vi "Juk3box_os.vi"() -> ()   [LabVIEW 2016]
uses:
  <vilib>/NXT/Block Support/NXT_InputPort.ctl
  <vilib>/NXT/Block Support/NXT_OutputPort.ctl
  <vilib>/NXT/Dual Mode Library/Sensors/Touch_Pressed.vi
  <vilib>/NXT/NXTIO Xnodes/NXTIONodeSubVIs/NXTMoveMotors.vi
  <vilib>/NXT/Dual Mode Library/Waits/Wait_Num.vi
  <vilib>/NXT/NXTIO Xnodes/NXTIONodeSubVIs/NXTStopMotors.vi
  <vilib>/NXT/Dual Mode Library/Sensors/EV3_Color_Color.vi
  <vilib>/NXT/NXTIO Xnodes/AddressXNode/NXTIOAddress.xnode
  <vilib>/NXT/NXTIO Xnodes/NXTIOXNode/NXTIO.xnode
  <vilib>/NXT/Subs/LVHSConnector.ctl
  <vilib>/NXT/LegoClasses/BrickReference/BrickReference.lvclass
panel:
  in  "Stop":bool
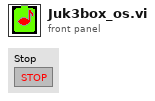
[diagram p1: front panel]
types:
  T1 = typedef "NXT_OutputPort.ctl" = u8
  T2 = typedef "NXT_InputPort.ctl" = u32
  T3 = typedef "LVHSConnector.ctl" = refnum<class "BrickReference.lvclass">
  T4 = typedef "ColorSensorColors.ctl" = enum16{"No Color", "Black", "Blue", "Green", "Yellow", "Red", "White", "Brown"}
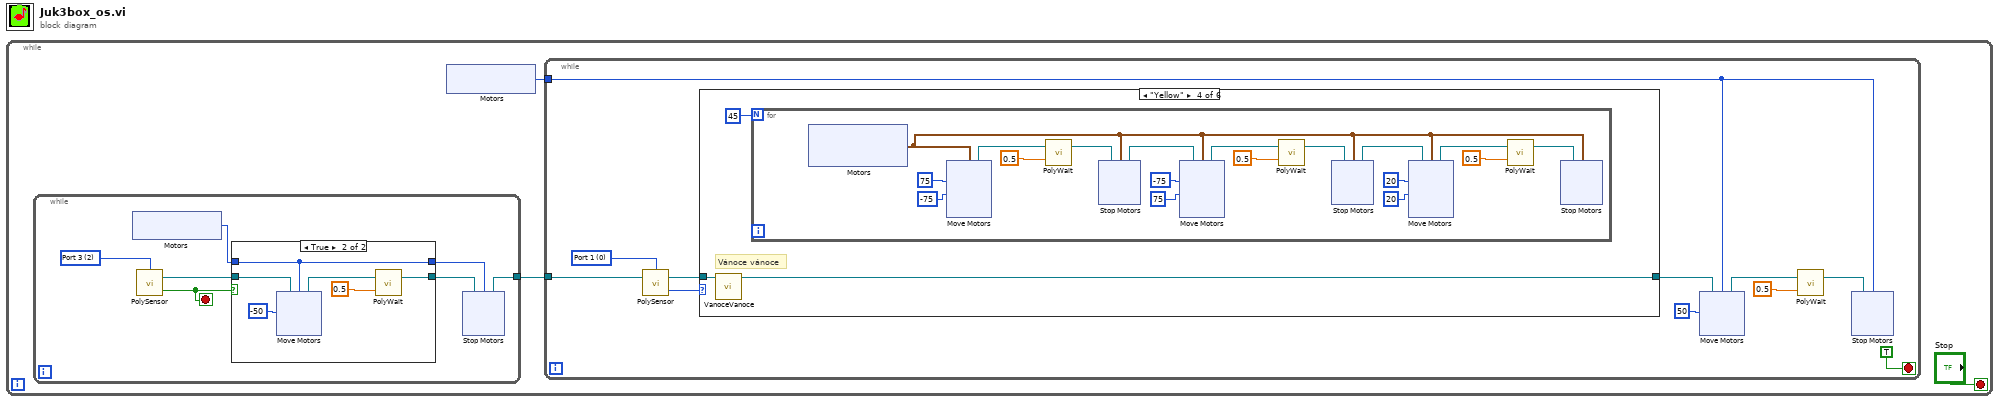
[diagram p0: block diagram]
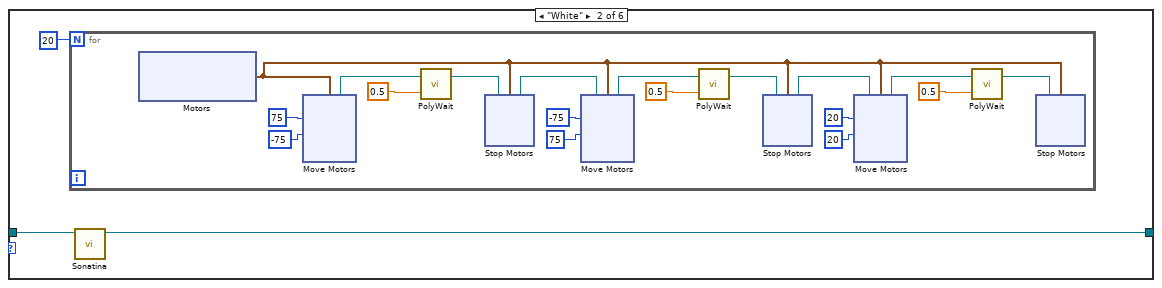
[diagram p3: hidden frame]
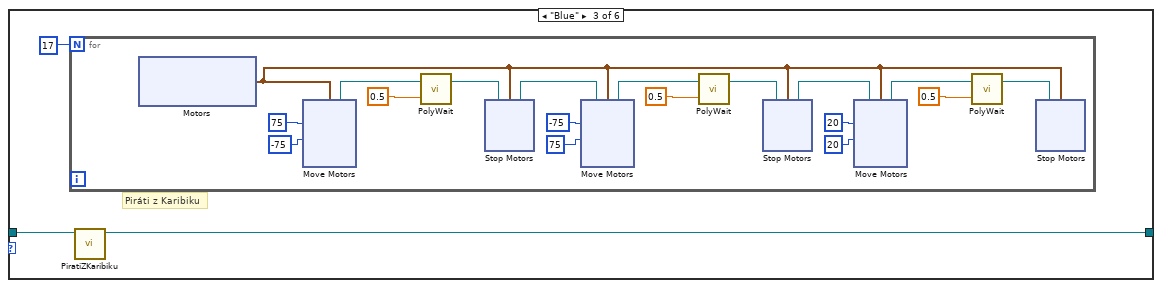
[diagram p4: hidden frame]
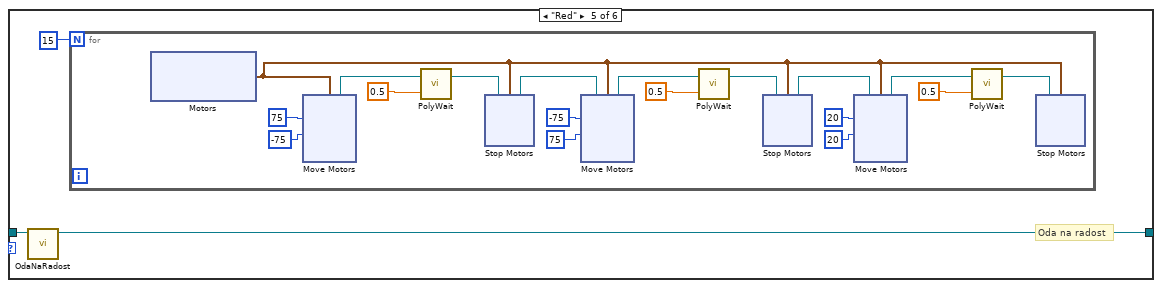
[diagram p5: hidden frame]
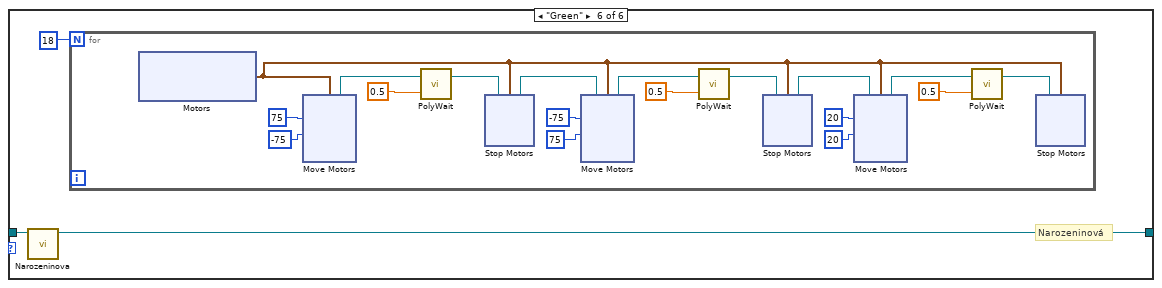
[diagram p6: hidden frame]
diagram:
  n1 = while {
    stop <- "Stop" stop-if-true
    n2 = while {
      tunnel: [w336] -> w2
      stop <- w334 stop-if-true
      w340 = T2 2 items=["Port 1", "Port 2", "Port 3", "Port 4"] ("Port (Port 1)")
      n3 = xnode "Motors"() -> ("Motor"=w339:T1)
      n4 = call-poly <vilib>:"PolySensor.vi"("Port (Port 1)"=w340) -> ("Yes / No"=w334:bool, "NXT/EV3"=w337:T3)  [unwired: 2 in]
      n5 = case shown="True" w334 {
        tunnel: w339 -> [w347 w349]
        tunnel: [w348 w351] -> w338
        tunnel: w337 -> [w348 w350]
        tunnel: [w347 w349] -> w335
        frame False {
        }
        frame True {
          n6 = xnode "Move Motors"("Power/Speed 1"=i8 -50, "Motors"=w349, "NXT/EV3"=w350) -> ("NXT/EV3"=w353:T3)
          n7 = call-poly <vilib>:"PolyWait.vi"("Time (1 sec)"=sgl 0.5, "NXT/EV3"=w353) -> ("NXT/EV3"=w351:T3)  [unwired: 2 in]
        }
      }
      n8 = xnode "Stop Motors"("Motors"=w335, "NXT/EV3"=w338) -> ("NXT/EV3"=w336:T3)
    }
    n9 = xnode "Motors"() -> ("Motor"=w3:T1)
    n10 = while {
      tunnel: w3 -> [w8]
      tunnel: w2 -> [w9]
      stop <- TRUE stop-if-true
      w14 = T2 0 items=["Port 1", "Port 2", "Port 3", "Port 4"] ("Port (Port 1)")
      n11 = call-poly <vilib>:"PolySensor.vi"("NXT/EV3"=w9, "Port (Port 1)"=w14) -> ("Detected Color"=w15:T4, "NXT/EV3"=w5:T3)  [unwired: 1 in]
      n12 = case shown="\"Yellow\"" w15 {
        tunnel: w5 -> [w28 w31 w91 w153 w214 w275]
        tunnel: [w28 w30 w92 w152 w213 w274] -> w10
        frame "No Color", Default {
        }
        frame "White" {
          n13 = for {
            N: 20 -> [_]
            n14 = xnode "Motors"() -> ("Motor"=w34:cluster{"Port":T1, "Port":T1})
            n15 = xnode "Move Motors"("Power/Speed 2"=i8 -75, "Power/Speed 1"=i8 75, "Motors"=w34) -> ("NXT/EV3"=w49:T3)  [unwired: 1 in]
            n16 = call-poly <vilib>:"PolyWait.vi"("Time (1 sec)"=sgl 0.5, "NXT/EV3"=w49) -> ("NXT/EV3"=w48:T3)  [unwired: 2 in]
            n17 = xnode "Stop Motors"("Motors"=w34, "NXT/EV3"=w48) -> ("NXT/EV3"=w40:T3)
            n18 = xnode "Move Motors"("Power/Speed 2"=i8 75, "Power/Speed 1"=i8 -75, "Motors"=w34, "NXT/EV3"=w40) -> ("NXT/EV3"=w41:T3)
            n19 = call-poly <vilib>:"PolyWait.vi"("Time (1 sec)"=sgl 0.5, "NXT/EV3"=w41) -> ("NXT/EV3"=w42:T3)  [unwired: 2 in]
            n20 = xnode "Stop Motors"("Motors"=w34, "NXT/EV3"=w42) -> ("NXT/EV3"=w33:T3)
            n21 = xnode "Move Motors"("Power/Speed 2"=i8 20, "Power/Speed 1"=i8 20, "Motors"=w34, "NXT/EV3"=w33) -> ("NXT/EV3"=w38:T3)
            n22 = call-poly <vilib>:"PolyWait.vi"("Time (1 sec)"=sgl 0.5, "NXT/EV3"=w38) -> ("NXT/EV3"=w37:T3)  [unwired: 2 in]
            n23 = xnode "Stop Motors"("Motors"=w34, "NXT/EV3"=w37) -> ()  [unwired: 1 out]
          }
          n24 = call "Sonatina.vi"("NXT/EV3"=w31) -> ("NXT/EV3 2"=w30:T3)  [unwired: 10 in]
        }
        frame "Blue" {
          # "Piráti z Karibiku"
          n25 = for {
            N: 17 -> [_]
            n26 = xnode "Motors"() -> ("Motor"=w95:cluster{"Port":T1, "Port":T1})
            n27 = xnode "Move Motors"("Power/Speed 2"=i8 -75, "Power/Speed 1"=i8 75, "Motors"=w95) -> ("NXT/EV3"=w110:T3)  [unwired: 1 in]
            n28 = call-poly <vilib>:"PolyWait.vi"("Time (1 sec)"=sgl 0.5, "NXT/EV3"=w110) -> ("NXT/EV3"=w109:T3)  [unwired: 2 in]
            n29 = xnode "Stop Motors"("Motors"=w95, "NXT/EV3"=w109) -> ("NXT/EV3"=w101:T3)
            n30 = xnode "Move Motors"("Power/Speed 2"=i8 75, "Power/Speed 1"=i8 -75, "Motors"=w95, "NXT/EV3"=w101) -> ("NXT/EV3"=w102:T3)
            n31 = call-poly <vilib>:"PolyWait.vi"("Time (1 sec)"=sgl 0.5, "NXT/EV3"=w102) -> ("NXT/EV3"=w103:T3)  [unwired: 2 in]
            n32 = xnode "Stop Motors"("Motors"=w95, "NXT/EV3"=w103) -> ("NXT/EV3"=w94:T3)
            n33 = xnode "Move Motors"("Power/Speed 2"=i8 20, "Power/Speed 1"=i8 20, "Motors"=w95, "NXT/EV3"=w94) -> ("NXT/EV3"=w99:T3)
            n34 = call-poly <vilib>:"PolyWait.vi"("Time (1 sec)"=sgl 0.5, "NXT/EV3"=w99) -> ("NXT/EV3"=w98:T3)  [unwired: 2 in]
            n35 = xnode "Stop Motors"("Motors"=w95, "NXT/EV3"=w98) -> ()  [unwired: 1 out]
          }
          n36 = call "PiratiZKaribiku.vi"("NXT/EV3"=w91) -> ("NXT/EV3 2"=w92:T3)  [unwired: 10 in]
        }
        frame "Yellow" {
          # "Vánoce vánoce"
          n37 = call "VanoceVanoce.vi"("NXT/EV3"=w153) -> ("NXT/EV3 2"=w152:T3)  [unwired: 10 in]
          n38 = for {
            N: 45 -> [_]
            n39 = xnode "Motors"() -> ("Motor"=w156:cluster{"Port":T1, "Port":T1})
            n40 = xnode "Move Motors"("Power/Speed 2"=i8 -75, "Power/Speed 1"=i8 75, "Motors"=w156) -> ("NXT/EV3"=w171:T3)  [unwired: 1 in]
            n41 = call-poly <vilib>:"PolyWait.vi"("Time (1 sec)"=sgl 0.5, "NXT/EV3"=w171) -> ("NXT/EV3"=w170:T3)  [unwired: 2 in]
            n42 = xnode "Stop Motors"("Motors"=w156, "NXT/EV3"=w170) -> ("NXT/EV3"=w162:T3)
            n43 = xnode "Move Motors"("Power/Speed 2"=i8 75, "Power/Speed 1"=i8 -75, "Motors"=w156, "NXT/EV3"=w162) -> ("NXT/EV3"=w163:T3)
            n44 = call-poly <vilib>:"PolyWait.vi"("Time (1 sec)"=sgl 0.5, "NXT/EV3"=w163) -> ("NXT/EV3"=w164:T3)  [unwired: 2 in]
            n45 = xnode "Stop Motors"("Motors"=w156, "NXT/EV3"=w164) -> ("NXT/EV3"=w155:T3)
            n46 = xnode "Move Motors"("Power/Speed 2"=i8 20, "Power/Speed 1"=i8 20, "Motors"=w156, "NXT/EV3"=w155) -> ("NXT/EV3"=w160:T3)
            n47 = call-poly <vilib>:"PolyWait.vi"("Time (1 sec)"=sgl 0.5, "NXT/EV3"=w160) -> ("NXT/EV3"=w159:T3)  [unwired: 2 in]
            n48 = xnode "Stop Motors"("Motors"=w156, "NXT/EV3"=w159) -> ()  [unwired: 1 out]
          }
        }
        frame "Red" {
          # "Oda na radost"
          n49 = call "OdaNaRadost.vi"("NXT/EV3"=w214) -> ("NXT/EV3 2"=w213:T3)  [unwired: 10 in]
          n50 = for {
            N: 15 -> [_]
            n51 = xnode "Motors"() -> ("Motor"=w218:cluster{"Port":T1, "Port":T1})
            n52 = xnode "Move Motors"("Power/Speed 2"=i8 -75, "Power/Speed 1"=i8 75, "Motors"=w218) -> ("NXT/EV3"=w232:T3)  [unwired: 1 in]
            n53 = call-poly <vilib>:"PolyWait.vi"("Time (1 sec)"=sgl 0.5, "NXT/EV3"=w232) -> ("NXT/EV3"=w231:T3)  [unwired: 2 in]
            n54 = xnode "Stop Motors"("Motors"=w218, "NXT/EV3"=w231) -> ("NXT/EV3"=w224:T3)
            n55 = xnode "Move Motors"("Power/Speed 2"=i8 75, "Power/Speed 1"=i8 -75, "Motors"=w218, "NXT/EV3"=w224) -> ("NXT/EV3"=w225:T3)
            n56 = call-poly <vilib>:"PolyWait.vi"("Time (1 sec)"=sgl 0.5, "NXT/EV3"=w225) -> ("NXT/EV3"=w226:T3)  [unwired: 2 in]
            n57 = xnode "Stop Motors"("Motors"=w218, "NXT/EV3"=w226) -> ("NXT/EV3"=w219:T3)
            n58 = xnode "Move Motors"("Power/Speed 2"=i8 20, "Power/Speed 1"=i8 20, "Motors"=w218, "NXT/EV3"=w219) -> ("NXT/EV3"=w223:T3)
            n59 = call-poly <vilib>:"PolyWait.vi"("Time (1 sec)"=sgl 0.5, "NXT/EV3"=w223) -> ("NXT/EV3"=w222:T3)  [unwired: 2 in]
            n60 = xnode "Stop Motors"("Motors"=w218, "NXT/EV3"=w222) -> ()  [unwired: 1 out]
          }
        }
        frame "Green" {
          # "Narozeninová"
          n61 = call "Narozeninova.vi"("NXT/EV3"=w275) -> ("NXT/EV3 2"=w274:T3)  [unwired: 10 in]
          n62 = for {
            N: 18 -> [_]
            n63 = xnode "Motors"() -> ("Motor"=w278:cluster{"Port":T1, "Port":T1})
            n64 = xnode "Move Motors"("Power/Speed 2"=i8 -75, "Power/Speed 1"=i8 75, "Motors"=w278) -> ("NXT/EV3"=w293:T3)  [unwired: 1 in]
            n65 = call-poly <vilib>:"PolyWait.vi"("Time (1 sec)"=sgl 0.5, "NXT/EV3"=w293) -> ("NXT/EV3"=w292:T3)  [unwired: 2 in]
            n66 = xnode "Stop Motors"("Motors"=w278, "NXT/EV3"=w292) -> ("NXT/EV3"=w284:T3)
            n67 = xnode "Move Motors"("Power/Speed 2"=i8 75, "Power/Speed 1"=i8 -75, "Motors"=w278, "NXT/EV3"=w284) -> ("NXT/EV3"=w285:T3)
            n68 = call-poly <vilib>:"PolyWait.vi"("Time (1 sec)"=sgl 0.5, "NXT/EV3"=w285) -> ("NXT/EV3"=w286:T3)  [unwired: 2 in]
            n69 = xnode "Stop Motors"("Motors"=w278, "NXT/EV3"=w286) -> ("NXT/EV3"=w277:T3)
            n70 = xnode "Move Motors"("Power/Speed 2"=i8 20, "Power/Speed 1"=i8 20, "Motors"=w278, "NXT/EV3"=w277) -> ("NXT/EV3"=w282:T3)
            n71 = call-poly <vilib>:"PolyWait.vi"("Time (1 sec)"=sgl 0.5, "NXT/EV3"=w282) -> ("NXT/EV3"=w281:T3)  [unwired: 2 in]
            n72 = xnode "Stop Motors"("Motors"=w278, "NXT/EV3"=w281) -> ()  [unwired: 1 out]
          }
        }
      }
      n73 = xnode "Move Motors"("Power/Speed 1"=i8 50, "Motors"=w8, "NXT/EV3"=w10) -> ("NXT/EV3"=w12:T3)
      n74 = call-poly <vilib>:"PolyWait.vi"("Time (1 sec)"=sgl 0.5, "NXT/EV3"=w12) -> ("NXT/EV3"=w7:T3)  [unwired: 2 in]
      n75 = xnode "Stop Motors"("Motors"=w8, "NXT/EV3"=w7) -> ()  [unwired: 1 out]
    }
  }
